vi "pp_writeCodesAutoPlay.vi"(0 "DAQmx Digital Out 1 In":refnum<k21>, 5 "Digital Out 1 Value":u8, 7 "DAQmx Digital Out 2 In":refnum<k21>, 9 "Digital Out 2 Value":u8, 11 "Error In":errorcluster) -> (4 "DAQmx Digital Out 1 Out":refnum<k21>, 8 "DAQmx Digital Out 2 Out":refnum<k21>, 15 "Error Out":errorcluster)   [LabVIEW 2013]
uses:
  <vilib>/DAQmx/write.llb/DAQmx Write (Digital U8 1Chan 1Samp).vi
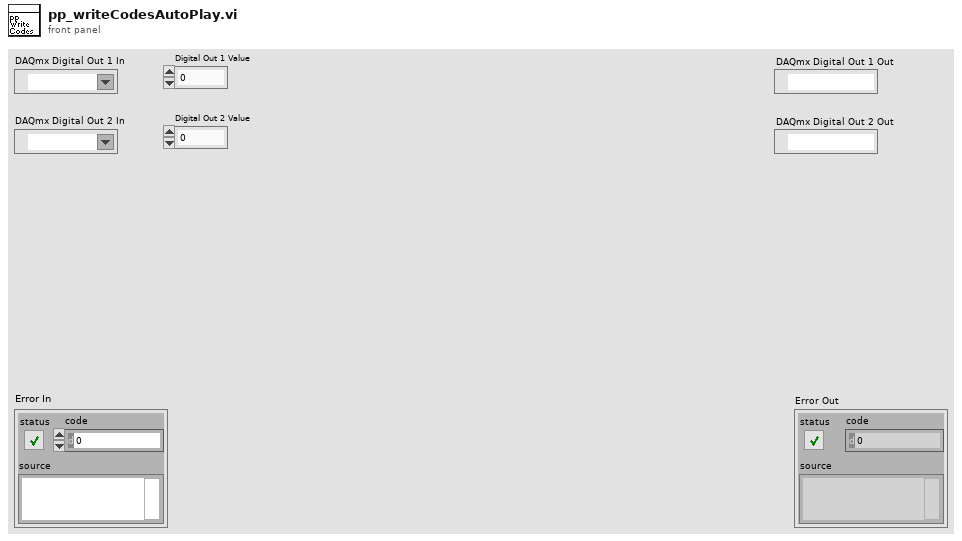
[diagram p1: front panel]
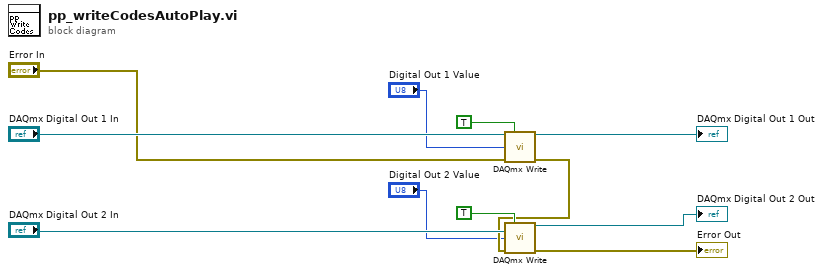
[diagram p0: block diagram]
diagram:
  n1 = call-poly <vilib>:"DAQmx Write.vi"("task/channels in"="DAQmx Digital Out 1 In", "auto start"=TRUE, "data"="Digital Out 1 Value", "error in"="Error In") -> ("task out"=→"DAQmx Digital Out 1 Out":refnum<k21>, "error out"=w6:errorcluster)  [unwired: 9 in, 1 out]
  n2 = call-poly <vilib>:"DAQmx Write.vi"("task/channels in"="DAQmx Digital Out 2 In", "auto start"=TRUE, "data"="Digital Out 2 Value", "error in"=w6) -> ("task out"=→"DAQmx Digital Out 2 Out":refnum<k21>, "error out"=→"Error Out":errorcluster)  [unwired: 9 in, 1 out]
